vi "WithinThresh.vi"(1 "Threshold":dbl, 2 "In":dbl) -> (0 "Within Thresh?":bool)   [LabVIEW 2013]
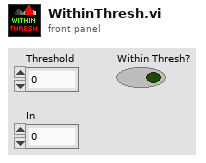
[diagram p1: front panel]
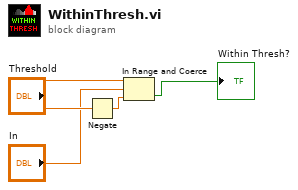
[diagram p0: block diagram]
diagram:
  n1 = Negate(x="Threshold") -> (-x=w2:dbl)
  n2 = In Range and Coerce(upper limit="Threshold", x="In", lower limit=w2) -> (In Range?=→"Within Thresh?":bool)  [unwired: 1 out]
